vi "SV TDMS Write Waveform Properties.vi"(0 "tdms file":refnum<k34>, 1 "array length":i32, 2 "dx":dbl, 3 "x0":dbl, 5 "group name":string, 7 "channel name":string, 11 "error in (no error)":errorcluster) -> (4 "tdms file out":refnum<k34>, 6 "group name out":string, 8 "channel name out":string, 15 "error out":errorcluster)   [LabVIEW 2017]
uses:
  <vilib>/addons/_NISVFA/_Shared subVIs/Controls/NI Channel Properties.ctl
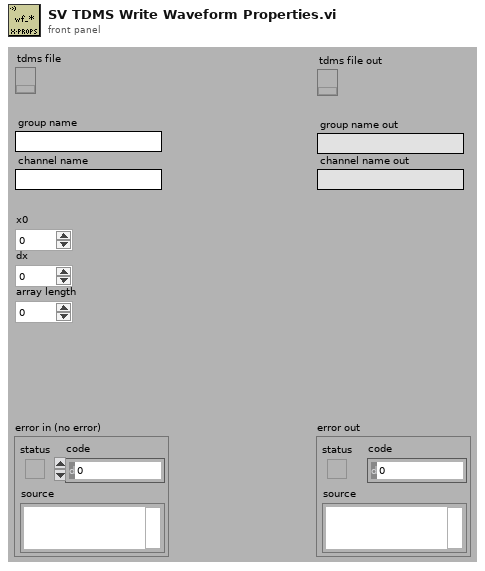
[diagram p1: front panel]
types:
  T1 = typedef "NI Channel Properties.ctl" = u16
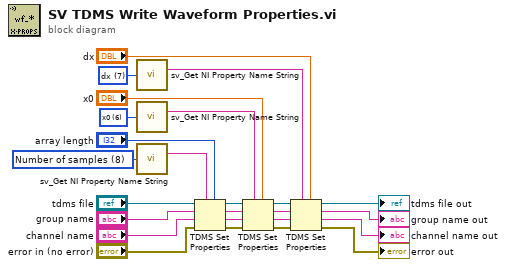
[diagram p0: block diagram]
diagram:
  w25 = T1 8 items=["Channel name", "Channel description", "Y-axis label", "Y-axis unit string", "X-axis label", "X-axis unit string", "x0", "dx", "Number of samples", "X channel", "Filter settled", "dB reference", "Window", "Window parameter", "Window size", "FFT size", "Peak units", "Spectrum type", "Magnitude scale", "Spectral density", "Sensor sensitivity (mV/EU)", "X-axis domain", "LabVIEW datatype"] ("property")
  w23 = T1 6 items=["Channel name", "Channel description", "Y-axis label", "Y-axis unit string", "X-axis label", "X-axis unit string", "x0", "dx", "Number of samples", "X channel", "Filter settled", "dB reference", "Window", "Window parameter", "Window size", "FFT size", "Peak units", "Spectrum type", "Magnitude scale", "Spectral density", "Sensor sensitivity (mV/EU)", "X-axis domain", "LabVIEW datatype"] ("property")
  w21 = T1 7 items=["Channel name", "Channel description", "Y-axis label", "Y-axis unit string", "X-axis label", "X-axis unit string", "x0", "dx", "Number of samples", "X channel", "Filter settled", "dB reference", "Window", "Window parameter", "Window size", "FFT size", "Peak units", "Spectrum type", "Magnitude scale", "Spectral density", "Sensor sensitivity (mV/EU)", "X-axis domain", "LabVIEW datatype"] ("property")
  n1 = call <vilib>:"sv_Get NI Property Name String.vi"("property"=w21) -> ("TDMS property name"=w20:string)  [unwired: 13 in, 1 out]
  n2 = call <vilib>:"sv_Get NI Property Name String.vi"("property"=w23) -> ("TDMS property name"=w22:string)  [unwired: 13 in, 1 out]
  n3 = call <vilib>:"sv_Get NI Property Name String.vi"("property"=w25) -> ("TDMS property name"=w24:string)  [unwired: 13 in, 1 out]
  n4 = TDMS Set Properties(5:"array length", 7:w24, 8:"error in (no error)", 9:"channel name", 10:"group name", 11:"tdms file") -> (0:w13:errorcluster, 1:w12:string, 2:w11:string, 3:w10:refnum<k34>)
  n5 = TDMS Set Properties(5:"x0", 7:w22, 8:w13, 9:w12, 10:w11, 11:w10) -> (0:w19:errorcluster, 1:w18:string, 2:w17:string, 3:w16:refnum<k34>)
  n6 = TDMS Set Properties(5:"dx", 7:w20, 8:w19, 9:w18, 10:w17, 11:w16) -> (0:→"error out":errorcluster, 1:→"channel name out":string, 2:→"group name out":string, 3:→"tdms file out":refnum<k34>)
